vi "AutoBike FPGA backup.vi"() -> ()   [LabVIEW 2016]
doc: "The roboRIO FPGA Shipping Personality. This personality supports:\n- 8 Analog Input channels with 1 sample\n- 2 Analog Output channels with 1 sample\n- 30 Digital I/O channels with 1 sample\n- 1 RSL channel\n- 4 Relay channels\n- 1 Button\n- 3 LEDs\n- 1 Accelerometer\n- 13 PWM channels\n- 6 Encoder channels\n- 2 SPI channels\n- 2 I2C channels\n- 2 UART channels\n- 1 CAN channel\n- 2 Analog Input Interrupt\n- 5 Digital Input Interrupt\n- 1 Timer Interrupt"
uses:
  Sub VIs/Utilities/Start Boolean.ctl
  <vilib>/Platform/TimedLoop/XDataNode/timing_clust.ctl
  <vilib>/Platform/TimedLoop/XDataNode/nitl_modes.ctl
  <vilib>/Platform/TimedLoop/XDataNode/wakeup.ctl
  <vilib>/rvi/Emulation/niFpgaGetClockAttributes.vi
  <vilib>/rvi/Emulation/niFpgaSctlEmulationGetInTimedLoop.vi
  <vilib>/rvi/Emulation/niFpgaEmulationReportErrorSimple.vi
  <vilib>/rvi/eio/common/nirviEmuTemplateMethod_errors.vi
  <vilib>/rvi/Emulation/niFpgaCriticalErrorInLSC.vi
  <vilib>/rvi/Emulation/niFpgaProcessEmulError.vi
  <vilib>/rvi/Emulation/niFpgaEmulationIsFPGAContextNoSignature.vi
  <vilib>/rvi/errors/niFpgaSetErrorForExecOnDevCompSimple.vi
  <vilib>/rvi/eio/common/nirviEmuReportErrorAndStop.vi
  <vilib>/rvi/DataTransferAndStorage/Container/Common/niFpgaContainerGetUniqueNameForEmu.vi
  <vilib>/rvi/FIFO/Fifo_Resource/nirvififoEmulationSetSize.vi
  <vilib>/rvi/FIFO/Fifo_Resource/nirviFifoEmulationQueueMgr.vi
  <instcachedir>/0/nirviFifoEmulationQueueMgr_E5CAEC123FF24DC58D834DCA3CDAA9B5.lvgen/nirviFifoEmulationQueueMgr_E5CAEC123FF24DC58D834DCA3CDAA9B5_002.vi
  <vilib>/Utility/error.llb/Clear Errors.vi
  <vilib>/rvi/FIFO/Fifo_Resource/nirvififoEmulationCreateLock.vi
  <vilib>/rvi/FIFO/Fifo_Resource/nirvififoEmulationObtainLock.vi
  <vilib>/rvi/FIFO/Fifo_Resource/nirvififoEmulationReleaseLock.vi
  <vilib>/rvi/occurrence/nirviWaitOnOccurrenceBase.vi
  <vilib>/rvi/errors/nirviReportUnexpectedCaseInternalError.vi
  <vilib>/rvi/errors/nirviReportUnexpectedCaseInternalError (U32).vi
  <vilib>/rvi/FIFO/Fifo_Resource/nirvififoEmulationDetermineInputValidOut.vi
  <vilib>/rvi/DataTransferAndStorage/Container/Common/niFpgaContainerSetEmuInfo.vi
  <vilib>/eio/EIONode/EIONode.xnode
  <vilib>/rvi/DataTransferAndStorage/Container/XNode/niFpgaContainer.xnode
  <vilib>/rvi/FIFO/Fifo_Resource/nirvififoEmulationRead.vi
  <vilib>/rvi/FIFO/Fifo_Resource/nirvififoEmulationWrite.vi
  <vilib>/Platform/TimedLoop/XDataNode/XDataNode.xnode
  <vilib>/rvi/LocalResourceManager/LocalResourceManager.xnode
  <vilib>/Platform/TimedLoop/XDataNode/XDNodeRunTimeDep.lvlib
panel:
  out "Position":i64
  in  "Stop encoder":bool
  in  "Reset counter":bool
  in  "Stop direction switch":bool
  in  "Switch direction":bool
  in  "Stop the walkassist mode":bool
  in  "Initiate walkassist mode":bool
  out "HallSensorValue":u8
  in  "Stop Hallsensor":bool
  out "dt":u32
  out "dt":u32
  out "DIO.SPI_CS3:0.IN":u8 format="%08b"
  in  "DIO.SPI_CS3:0.DIR":u8 format="%08b"
  in  "DIO.SPI_CS3:0.OUT":u8 format="%08b"
  in  "IRQ.TIMER.SETTIME":T1
  in  "IRQ.TIMER.WRITE":u32
  out "IRQ.TIMER.READ":u32
  in  "IRQ.DI_BTN.NO":u8
  in  "IRQ.DI_BTN.CNT":u32
  in  "IRQ.DI_BTN.FALL":bool
  in  "IRQ.DI_BTN.RISE":bool
  in  "IRQ.DI_BTN.ENA":bool
  in  "IRQ.AI_B_0.HYSTERESIS":u16=17
  in  "IRQ.AI_B_1.HYSTERESIS":u16=17
  in  "IRQ.AI_B_1.NO":u8
  in  "IRQ.AI_B_0.NO":u8
  in  "IRQ.AI_B_1.THRESHOLD":u16
  in  "IRQ.AI_B_0.THRESHOLD":u16
  in  "IRQ.AI_B_3:0.CNFG":u8 format="%.0b"
  in  "IRQ.DIO_B_0.NO":u8
  in  "IRQ.DIO_B_1.NO":u8
  in  "IRQ.DIO_B_2.NO":u8
  in  "IRQ.DIO_B_3.NO":u8
  in  "IRQ.DIO_B_3.CNT":u32
  in  "IRQ.DIO_B_2.CNT":u32
  in  "IRQ.DIO_B_1.CNT":u32
  in  "IRQ.DIO_B_0.CNT":u32
  in  "IRQ.DIO_B_7:0.FALL":u8 format="%08b"
  in  "IRQ.DIO_B_7:0.RISE":u8 format="%08b"
  in  "IRQ.DIO_B_7:0.ENA":u8 format="%08b"
  in  "SPI.SPI.IRQ.NO":u8=15
  in  "SPI.B.IRQ.NO":u8=15
  out "DIO.DIO_9:8.IN":u8 format="%08b"
  in  "ENC.DIO_3.CNFG":u8 format="%08b"
  out "ENC.DIO_3.CNTR":u32
  out "ENC.DIO_3.STAT":u8 format="%08b"
  in  "ENC.DIO_4.CNFG":u8 format="%08b"
  out "ENC.DIO_4.CNTR":u32
  out "ENC.DIO_4.STAT":u8 format="%08b"
  in  "DIO.DIO_9:8.OUT":u8 format="%08b"
  in  "DIO.DIO_9:8.DIR":u8 format="%08b"
  in  "ENC.DIO_2.CNFG":u8 format="%08b"
  out "ENC.DIO_2.CNTR":u32
  out "ENC.DIO_2.STAT":u8 format="%08b"
  out "ENC.DIO_1.STAT":u8 format="%08b"
  out "ENC.DIO_1.CNTR":u32
  in  "ENC.DIO_1.CNFG":u8 format="%08b"
  out "DIO.DIO_7:0.IN":u8 format="%08b"
  in  "SYS.SELECTDIO":u8 format="%08b"
  in  "DIO.DIO_7:0.DIR":u8 format="%08b"
  in  "DIO.DIO_7:0.OUT":u8 format="%08b"
  out "ENC.DIO_0.STAT":u8 format="%08b"
  out "ENC.DIO_0.CNTR":u32
  in  "ENC.DIO_0.CNFG":u8 format="%08b"
  out "DI.BTN":u8 format="%08b"
  in  "DO.LED 5:0":u8 format="%06b"
  in  "DO.RSL.OUT":bool
  out "SPI.SPI.STAT":u8 format="%08b"
  in  "SPI.SPI.GO":T1
  in  "SPI.SPI.CNT":u16
  in  "SPI.SPI.CNFG":u16 format="%016b"
  out "SPI.SPI.DATI":u16
  in  "SPI.SPI.DATO":u16
  out "I2C.I2C.DATI":u8
  out "I2C.I2C.STAT":u8 format="%08b"
  in  "I2C.I2C.DATO":u8
  in  "I2C.I2CADDR":u8 format="%08b"
  in  "I2C.I2C.CNTR":u8
  in  "I2C.I2C.CNTL":u8 format="%08b"
  in  "I2C.I2C.CNFG":u8 format="%08b"
  in  "I2C.I2C.GO":T1
  out "ACC.Z.VAL":u16
  out "ACC.Y.VAL":u16
  out "ACC.X.VAL":u16
  in  "DO.RELAY.OUT":u8 format="%08b"
  out "SYS.ACC.RDY":bool
  out "SYS.RDY":bool
  in  "PWM.PWM_5.MAX":u16
  in  "PWM.PWM_5.CMP":u16
  in  "PWM.PWM_5.CNFG":u8 format="%08b"
  in  "PWM.PWM_5.CS":u8
  out "PWM.PWM_5.CNTR":u16
  in  "PWM.PWM_6.MAX":u16
  in  "PWM.PWM_6.CMP":u16
  in  "PWM.PWM_6.CNFG":u8 format="%08b"
  in  "PWM.PWM_6.CS":u8
  out "PWM.PWM_6.CNTR":u16
  in  "PWM.PWM_7.MAX":u16
  in  "PWM.PWM_7.CMP":u16
  in  "PWM.PWM_7.CNFG":u8 format="%08b"
  in  "PWM.PWM_7.CS":u8
  out "PWM.PWM_7.CNTR":u16
  in  "PWM.PWM_8.MAX":u16
  in  "PWM.PWM_8.CMP":u16
  in  "PWM.PWM_8.CNFG":u8 format="%08b"
  in  "PWM.PWM_8.CS":u8
  out "PWM.PWM_8.CNTR":u16
  in  "PWM.PWM_9.MAX":u16
  in  "PWM.PWM_9.CMP":u16
  in  "PWM.PWM_9.CNFG":u8 format="%08b"
  in  "PWM.PWM_9.CS":u8
  out "PWM.PWM_9.CNTR":u16
  in  "PWM.PWM_4.MAX":u16
  in  "PWM.PWM_4.CMP":u16
  in  "PWM.PWM_4.CNFG":u8 format="%08b"
  in  "PWM.PWM_4.CS":u8
  out "PWM.PWM_4.CNTR":u16
  in  "PWM.PWM_3.MAX":u16
  in  "PWM.PWM_3.CMP":u16
  in  "PWM.PWM_3.CNFG":u8 format="%08b"
  in  "PWM.PWM_3.CS":u8
  out "PWM.PWM_3.CNTR":u16
  in  "PWM.PWM_2.MAX":u16
  in  "PWM.PWM_2.CMP":u16
  in  "PWM.PWM_2.CNFG":u8 format="%08b"
  in  "PWM.PWM_2.CS":u8
  out "PWM.PWM_2.CNTR":u16
  in  "PWM.PWM_1.MAX":u16
  in  "PWM.PWM_1.CMP":u16
  in  "PWM.PWM_1.CNFG":u8 format="%08b"
  in  "PWM.PWM_1.CS":u8
  out "PWM.PWM_1.CNTR":u16
  out "PWM.PWM_0.CNTR":u16
  in  "PWM.PWM_0.CS":u8
  in  "PWM.PWM_0.CNFG":u8 format="%08b"
  in  "PWM.PWM_0.CMP":u16
  in  "PWM.PWM_0.MAX":u16
  in  "AO.B_0.VAL":u16
  in  "AO.B_1.VAL":u16
  in  "AO.SYS.GO":T1
  out "AO.SYS.STAT":bool
  out "AI.B_0.VAL":u16
  out "AI.B_1.VAL":u16
  out "AI.B_2.VAL":u16
  out "AI.B_3.VAL":u16
  out "AI.AI_0.VAL":u16
  out "AI.AI_1.VAL":u16
  out "AI.AI_2.VAL":u16
  out "AI.AI_3.VAL":u16
  out "SYS.AI.RDY":bool
  in  "SYS.SELECTB":u8 format="%08b"
  in  "DIO.B_7:0.OUT":u8 format="%08b"
  in  "DIO.B_7:0.DIR":u8 format="%08b"
  out "DIO.B_7:0.IN":u8 format="%08b"
  in  "DIO.B_15:8.OUT":u8 format="%08b"
  in  "DIO.B_15:8.DIR":u8 format="%08b"
  out "DIO.B_15:8.IN":u8 format="%08b"
  in  "SPI.B.DATO":u16
  out "SPI.B.DATI":u16
  in  "SPI.B.CNFG":u16 format="%016b"
  in  "SPI.B.CNT":u16
  in  "SPI.B.GO":T1
  out "SPI.B.STAT":u8 format="%08b"
  in  "PWM.B_0.MAX":u16
  in  "PWM.B_0.CMP":u16
  in  "PWM.B_0.CNFG":u8 format="%08b"
  in  "PWM.B_0.CS":u8
  out "PWM.B_0.CNTR":u16
  in  "PWM.B_1.CMP":u16
  in  "PWM.B_1.MAX":u16
  out "PWM.B_1.CNTR":u16
  in  "PWM.B_1.CNFG":u8 format="%08b"
  in  "PWM.B_1.CS":u8
  in  "PWM.B_2.CMP":u16
  in  "PWM.B_2.MAX":u16
  out "PWM.B_2.CNTR":u16
  in  "PWM.B_2.CNFG":u8 format="%08b"
  in  "PWM.B_2.CS":u8
  in  "I2C.B.DATO":u8
  out "I2C.B.DATI":u8
  in  "I2C.B.ADDR":u8 format="%08b"
  in  "I2C.B.CNTR":u8
  in  "I2C.B.CNTL":u8 format="%08b"
  out "I2C.B.STAT":u8 format="%08b"
  in  "I2C.B.CNFG":u8 format="%08b"
  in  "I2C.B.GO":T1
  in  "ENC.B.CNFG":u8 format="%08b"
  out "ENC.B.CNTR":u32
  out "ENC.B.STAT":u8 format="%08b"
  # "System"
  # "Onboard Devices"
  # "Connector B"
  # "DIO"
  # "SPI"
  # "PWM"
  # "I2C"
  # "AI"
  # "RELAY"
  # "RSL"
  # "Accelerometer"
  # "SPI Master"
  # "Analog Input"
  # "Analog Output"
  # "Digital I/O"
  # "Counters / PWM"
  # "Digital I/O"
  # "Encoders"
  # "IO Configuration"
  # "Buttons & LEDs"
  # "SPI CS DIO"
  # "Analog Interrupt"
  # "Digital Interrupt"
  # "Encoders"
  # "IO Configuration"
  # "Button Interrupt"
  # "I2C Master"
  # "FPGA Timer"
  # "This VI contains the default FPGA personality in addition to code that generates a sine waveform and filtered sine waveform based on parameters set by RT Main.vi. Keeping the default personality allows you to continue using the roboRIO APIs even after adding custom FPGA code."
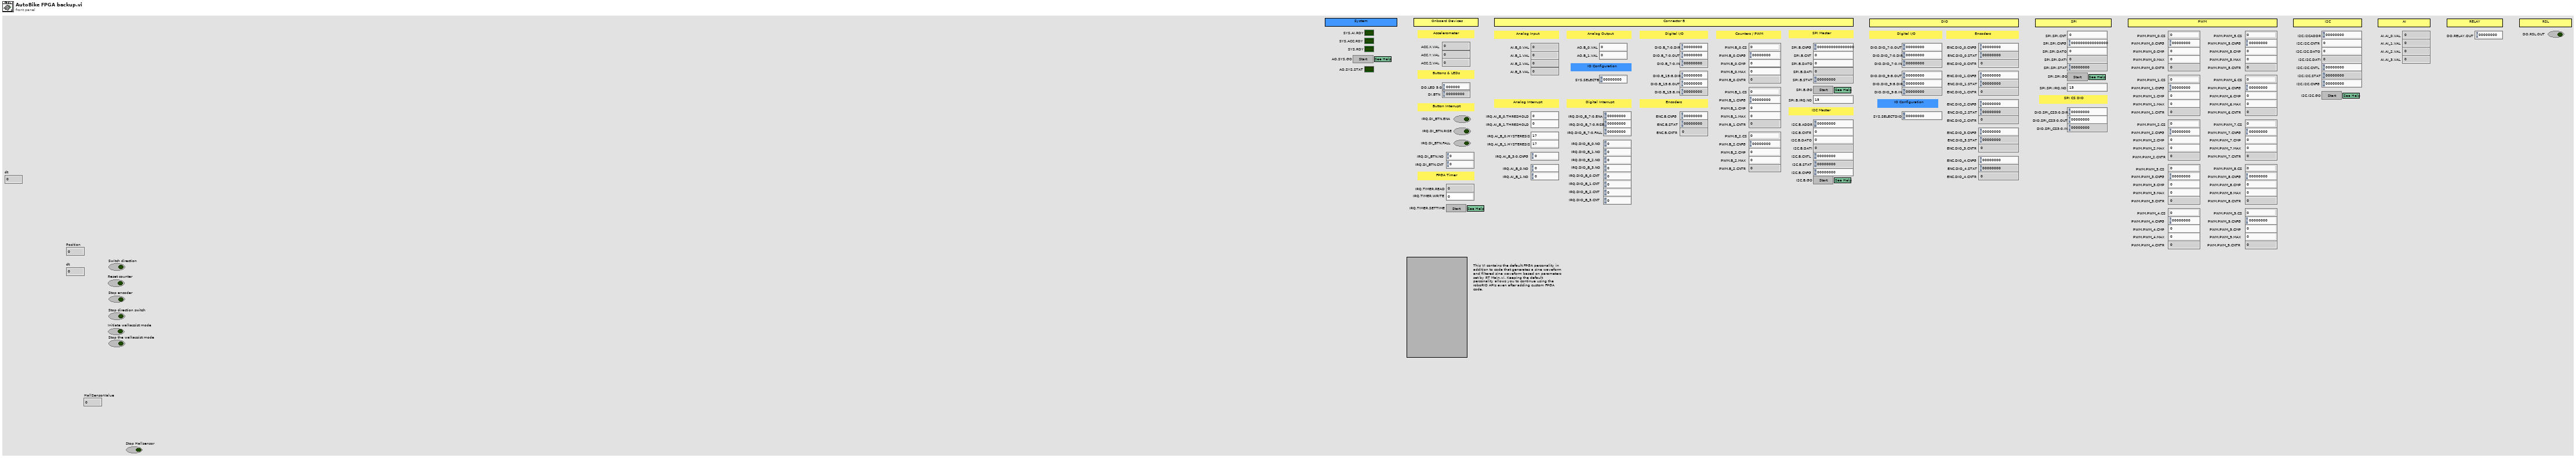
[diagram p1: front panel]
types:
  T1 = typedef "Start Boolean.ctl" = bool
  T2 = typedef "XDNodeRunTimeDep.lvlib/timing_clust.ctl" = cluster{"Expected End [f-1]":u64, "Actual End [f-1]":u64, "Finished Late? [f-1]":bool, "Expected End [i-1]":u64, "Actual End [i-1]":u64, "Finished Late? [i-1]":bool, "Expected Start [i]":u64, "Actual Start [i]":u64, "Expected Start [f]":u64, "Actual Start [f]":u64, "Source Name":string, "Structure Name":string, "Period":i64, "Deadline":i64, "Offset":i64, "Start":i64, "Priority":i32, "Timeout":i32, "Mode":T3, "Wakeup Reason":T4, "Error":errorcluster, "Source Type":string, "Secondary Source Type":string, "Global End Time":u64, "Global Start Time":u64, "Frame Duration":u64, "Iteration Duration":u64, "Assigned CPU":i32, "I/O Scan Engine Mode":u32}
  T3 = typedef "XDNodeRunTimeDep.lvlib/nitl_modes.ctl" = enum32{"No Change", "Process missed periods, maintain original phase", "Discard missed periods, maintain original phase", "Process missed periods, ignore original phase", "Discard missed periods, ignore original phase"}
  T4 = typedef "XDNodeRunTimeDep.lvlib/wakeup.ctl" = enum32{"Normal", "Aborted", "Asynchronous wakeup", "Timing source error", "Timed loop error", "Timeout"}
diagram:
  # "The accelerometer nodes take some time before the FPGA can first read the values. This is because it takes time to read from the accelerometer. An iteration of the While Loop will not complete until the accelerometer values have been read.\n\nAfter the completion of the first iteration of the While Loop, all indicators have valid values."
  # "The analog output nodes take some time before the FPGA write the values to the pins. The GO and STAT registers are used to handshake between the FPGA and host. When the host wants the values to be written, the host sets the GO register to TRUE. If the host reads the STAT register before setting the value of the GO register, it can wait for the value of the STAT register to invert. The value inversion tells the host that the output values have been written."
  # "The FPGA timer fires the interrupt request (IRQ) when TIMER.Read counts down to zero. If TIMER.Read is not zero, it counts down to one per microsecond."
  # "The analog input nodes take some time before the FPGA can first read the values. This is because it takes time to set up the Analog-to-Digital converter (ADC) and convert the first reading. An iteration of the While Loop will not complete until all the analog input channels have been sampled.\n\nAfter the completion of the first iteration of the While Loop, all indicators have valid values."
  # "Note: On some hardware a \"ghosting effect\" may occur on any unconnected AI channels. For example, if channel AI0 is connected and channels AI1~AI7 are not connected the the value read at AI0 may be seen on indicators AI1~AI7. This is common for hardware that use a multiplexed (MUXed) Analog-to-Digital converter (ADC), because the input analog signal is used to charge a capacitor which does not discharge before the unconnected channel is read.\n\nYou can hide the \"ghosting effect\" by using an mask register. This register is used to decide when the indicator should be updated."
  # "The only interface that sends interrupts to the RT side. Timer interrupts, analog input interrupts, digital input interrupts, and SPI interrupt share this interface.\n\nAll interrupts work in sequence. One interrupt waits until the previous interrupt request (IRQ) gets acknowledged on the RT side."
  # "NOTE: The SYS.RDY boolean MUST exist and must become TRUE at some point otherwise the myRIO API will not function correctly."
  # "There is some delay between when the FPGA code starts and the analog inputs, accelerometer, and scaling values outputs are valid. If the host wants to ensure that there are valid values in theses registers it should wait for each subsystem to finish its initialization process. \n\nWhen all subsystems have finished initializinig, the SYS.RDY indicator will be true, which can be polled by the host to determine the status of the FPGA. Alternatively, the host can poll the individual SYS.xx.RDY indicators to determine the status of the individual subsystems.\n\nThis loop continues indefinitely, essentially making SYS.RDY a read-only register."
  n1 = flat-sequence {
    tunnel: [i64 0] -> w3
    tunnel: [FALSE ("DIO/DIO3")] -> w2
    tunnel: [u8 0] -> w1
    tunnel: w3 -> [w34]
    tunnel: w2 -> [w33]
    tunnel: w1 -> [w28]
    frame #0 {
      # "Initialise"
    }
    frame #1 {
      n2 = while {
        shift-right: [w52] -> _
        shift-left: w33 -> [w56]
        tunnel: w28 -> [w49]
        stop <- "Stop Hallsensor" stop-if-true
        n3 = node-c288() -> (w51:T2)  [unwired: 1 in]
        n4 = call "Tick Count4"() -> ("Tick Count(uSec)"=w55:u32)
        n5 = timed-loop {
          shift-right: [w62] -> _
          shift-left: w49 -> [w73]
          tunnel: w55 -> [w71]
          shift-right: [w69] -> w52
          shift-left: w56 -> [w74]
          tunnel: [w72] -> w58
          tunnel: [w71] -> w57
          timing: w51 -> [_]
          timing-out: [_] -> w50
          i -> [w60]
          stop <- w61 stop-if-true
          # "Calculates the time it takes to collect 4 rises, i.e one revolution of the wheel"
          # "If A is high and we have a change we \nshould increament the counter"
          # "Reads the output from the hallsensor and outputs the number of change in rises"
          # "Hallsensor counter"
          n6 = call "Tick Count3"() -> ("Tick Count(uSec)"=w72:u32)
          n7 = xnode "FPGA I/O Node"() -> ("DIO/DIO3"=w69:bool)  [unwired: 1 in, 1 out]
          n8 = Equal To 0?(x=w60) -> (x = 0?=w59:bool)
          n9 = Exclusive Or(1:w74, 2:w69) -> (0:w67:bool)
          n10 = Select(t=u8 0, s=w59, f=w73) -> (s? t:f=w64:u8)
          n11 = And(x=w69, y=TRUE) -> (x .and. y?=w68:bool)
          n12 = And(x=w68, y=w67) -> (x .and. y?=w66:bool)
          n13 = Increment(x=w64) -> (x+1=w65:u8)
          n14 = Select(t=w65, s=w66, f=w64) -> (s? t:f=w62:u8)
          "HallSensorValue" <- w62
          n15 = Equal?(x=u8 4, y=w62) -> (x = y?=w61:bool)
        }
        n16 = node-c288(w50) -> ()
        n17 = Subtract(x=w58, y=w57) -> (x-y=→"dt":u32)
      }
      n18 = node-c288() -> (w30:T2)  [unwired: 1 in]
      n19 = node-c288() -> (w36:T2)  [unwired: 1 in]
      n20 = timed-loop {
        timing: w30 -> [_]
        timing-out: [_] -> w29
        stop <- "Stop the walkassist mode" stop-if-true
        # "Put the bike in walk assist."
        # "Walkassist"
        n21 = xnode "FPGA I/O Node"("DIO/DIO2"="Initiate walkassist mode") -> ()  [unwired: 1 in, 1 out]
      }
      n22 = timed-loop {
        shift-right: [w90] -> _
        shift-left: w34 -> [w81]
        shift-right: [w87] -> _
        shift-left: _ -> [w85]
        shift-right: [w86] -> _
        shift-left: _ -> [w84]
        timing: w36 -> [_]
        timing-out: [_] -> w35
        stop <- "Stop encoder" stop-if-true
        # "Decoder, reads both signals and check if there is any change to any of the channels, if there is a change current A channel\nis compared to previous B channel to determine which direction the motor is going and updates the position counter\naccordingly. The counter is resetted each time the Main VI is deployed."
        # "Motor Decoder"
        n23 = xnode "FPGA I/O Node"() -> ("DIO/DIO7"=w87:bool, "DIO/DIO8"=w86:bool)  [unwired: 2 in, 2 out]
        n24 = Exclusive Or(1:w84, 2:w87) -> (0:w83:bool)
        n25 = Select(t=i64 0, s="Reset counter", f=w81) -> (s? t:f=w89:i64)
        n26 = Exclusive Or(1:w85, 2:w87) -> (0:w97:bool)
        n27 = Exclusive Or(1:w84, 2:w86) -> (0:w96:bool)
        n28 = Or(x=w97, y=w96) -> (x .or. y?=w82:bool)
        n29 = Select(t=i64 1, s=w83, f=i64 -1) -> (s? t:f=w92:i64)
        n30 = Add(x=w92, y=w89) -> (x+y=w91:i64)
        n31 = Select(t=w91, s=w82, f=w89) -> (s? t:f=w90:i64)
        "Position" <- w90
      }
      n32 = node-c288(w29) -> ()
      n33 = node-c288() -> (w32:T2)  [unwired: 1 in]
      n34 = timed-loop {
        timing: w32 -> [_]
        timing-out: [_] -> w31
        stop <- "Stop direction switch" stop-if-true
        # "Switch the direction of the steering\nmotor."
        # "Switch direction"
        n35 = xnode "FPGA I/O Node"("DIO/DIO9"="Switch direction") -> ()  [unwired: 1 in, 1 out]
      }
      n36 = node-c288(w31) -> ()
      n37 = node-c288(w35) -> ()
    }
  }
  n38 = while {
    stop <- FALSE stop-if-true
    # "Host Synchronization"
    n39 = local read "SYS.ACC.RDY"() -> (w103:bool)
    n40 = local read "SYS.AI.RDY"() -> (w105:bool)
    n41 = Compound Arithmetic op=AND(w105, w103) -> (→"SYS.RDY":bool)
  }
  n42 = while {
    stop <- FALSE stop-if-true
    # "Interrupt to RT"
    n43 = xnode ("FIFO Method Node")("Timeout"=-1) -> ("Element"=w108:u8)  [unwired: 1 in, 2 out]
    n44 = call <vilib>:"niFPGA Interrupt.vi"("Wait Until Cleared (F)"=TRUE, "IRQ Number (0)"=w108) -> ()  [unwired: 1 in]
  }
  n45 = while {
    stop <- FALSE stop-if-true
    # "Timer"
    n46 = local read "IRQ.TIMER.READ"() -> (w113:u32)
    n47 = Select(t="IRQ.TIMER.WRITE", s="IRQ.TIMER.SETTIME", f=w113) -> (s? t:f=w111:u32)
    n48 = case shown="Default" w111 {
      selector: w111 -> [w117 w120]
      tunnel: [w117 w118] -> w110
      frame 0 {
      }
      frame Default {
        n49 = Decrement(x=w120) -> (x-1=w119:u32)
        n50 = case shown="0" w119 {
          selector: w119 -> [w121 w124]
          tunnel: [w121 w124] -> w118
          frame Default {
          }
          frame 0 {
            w123 = u8 0  # Reserved for Timer IRQ
            n51 = xnode ("FIFO Method Node")("Element"=w123, "Timeout"=-1) -> ()  [unwired: 1 in, 2 out]
          }
        }
      }
    }
    "IRQ.TIMER.READ" <- w110
    n52 = call "Loop Timer"("Count(uSec)"=u8 1 ("Count(mSec)")) -> ()  [unwired: 1 out]
  }
  n53 = xnode "VI-Defined FIFO Configuration"() -> ("FIFO Out"=w5:refnum<k21>)
  n54 = while {
    tunnel: w5 -> [w133]
    i -> [w147]
    stop <- FALSE stop-if-true
    # "Analog Input"
    n55 = Greater Than 0?(x=w147) -> (x > 0?=→"SYS.AI.RDY":bool)
    n56 = xnode "FPGA I/O Node"() -> ("MXP/AI0"=w126:u16, "MXP/AI1"=w125:u16, "MXP/AI2"=→"AI.B_2.VAL":u16, "MXP/AI3"=→"AI.B_3.VAL":u16, "AnalogIn0"=→"AI.AI_0.VAL":u16, "AnalogIn1"=→"AI.AI_1.VAL":u16, "AnalogIn2"=→"AI.AI_2.VAL":u16, "AnalogIn3"=→"AI.AI_3.VAL":u16)  [unwired: 8 in, 8 out]
    "AI.B_0.VAL" <- w126
    "AI.B_1.VAL" <- w125
    n57 = Number To Boolean Array(number="IRQ.AI_B_3:0.CNFG") -> (Boolean array=w134:bool[])
    n58 = Index Array(array=w134) -> (element #1=w136:bool, element #2=w137:bool, element #3=w139:bool, element #4=w140:bool)  [unwired: 4 in]
    n59 = call "Check AI IRQ.vi"("Hysteresis"="IRQ.AI_B_1.HYSTERESIS", "FIFO In"=w133, "IRQ Number"="IRQ.AI_B_1.NO", "Threshold"="IRQ.AI_B_1.THRESHOLD", "Analog Value"=w125, "Rising Edge?"=w140, "Enable Interrupt?"=w139) -> ()  [unwired: 5 in]
    n60 = call "Check AI IRQ.vi"("Hysteresis"="IRQ.AI_B_0.HYSTERESIS", "FIFO In"=w133, "IRQ Number"="IRQ.AI_B_0.NO", "Threshold"="IRQ.AI_B_0.THRESHOLD", "Analog Value"=w126, "Rising Edge?"=w137, "Enable Interrupt?"=w136) -> ()  [unwired: 5 in]
  }
  n61 = while {
    stop <- FALSE stop-if-true
    # "Analog Output"
    n62 = feedback #1(FALSE) -> (w151:bool)
    n63 = case shown="True" "AO.SYS.GO" {
      tunnel: "AO.B_0.VAL" -> [_ w161]
      tunnel: "AO.B_1.VAL" -> [_ w160]
      tunnel: w151 -> [w156 w159]
      tunnel: [w156 w157] -> w149
      frame False {
      }
      frame True {
        n64 = flat-sequence {
          tunnel: w161 -> [w164]
          tunnel: w160 -> [w163]
          tunnel: w159 -> [w162]
          tunnel: [w162] -> w158
          tunnel: w158 -> [w166]
          tunnel: [w165] -> w157
          frame #0 {
            n65 = xnode "FPGA I/O Node"("MXP/AO0"=w164, "MXP/AO1"=w163) -> ()  [unwired: 2 in, 2 out]
          }
          frame #1 {
            n66 = Not(x=w166) -> (.not. x?=w165:bool)
          }
        }
      }
    }
    "AO.SYS.STAT" <- w149
    n67 = feedback-in #1(w149) -> ()
  }
  n68 = while {
    i -> [w174]
    stop <- FALSE stop-if-true
    # "Onboard Accelerometer"
    n69 = xnode "FPGA I/O Node"() -> ("AccelerationX"=w172:i16, "AccelerationY"=w171:i16, "AccelerationZ"=w170:i16)  [unwired: 3 in, 3 out]
    n70 = Greater Than 0?(x=w174) -> (x > 0?=→"SYS.ACC.RDY":bool)
    n71 = To Unsigned Word Integer(number=w172) -> (unsigned 16bit integer=→"ACC.X.VAL":u16)
    n72 = To Unsigned Word Integer(number=w171) -> (unsigned 16bit integer=→"ACC.Y.VAL":u16)
    n73 = To Unsigned Word Integer(number=w170) -> (unsigned 16bit integer=→"ACC.Z.VAL":u16)
  }
  n74 = xnode "VI-Defined FIFO Configuration"() -> ("FIFO Out"=w4:refnum<k21>)
  n75 = node-c288() -> (w10:T2)  [unwired: 1 in]
  n76 = timed-loop {
    timing: w10 -> [_]
    timing-out: [_] -> w9
    tunnel: w4 -> [w181]
    stop <- FALSE stop-if-true
    # "Button IRQ"
    # "Onboard DIO"
    n77 = xnode "FPGA I/O Node"() -> ("User Button"=w182:bool)  [unwired: 1 in, 1 out]
    n78 = Number To Boolean Array(number="DO.LED 5:0") -> (Boolean array=w192:bool[])
    n79 = Index Array(array=w192) -> (element #1=w190:bool, element #2=w189:bool, element #3=w188:bool, element #4=w187:bool, element #5=w186:bool, element #6=w185:bool)  [unwired: 6 in]
    n80 = Build Array(w182) -> (w184:bool[])
    n81 = call "DIO IRQ 1-bit.vi"("IRQ.NO"="IRQ.DI_BTN.NO", "IRQ.CNT"="IRQ.DI_BTN.CNT", "FIFO in"=w181, "IRQ.FALL"="IRQ.DI_BTN.FALL", "IRQ.RISE"="IRQ.DI_BTN.RISE", "IRQ.ENA"="IRQ.DI_BTN.ENA", "DIO"=w182) -> ()  [unwired: 5 in]
    n82 = Boolean Array To Number(Boolean array=w184) -> (number=→"DI.BTN":u8)
    n83 = xnode "FPGA I/O Node"("Radio LED Green"=w190, "Radio LED Red"=w189, "Comm LED Green"=w188, "Comm LED Red"=w187, "Mode LED Green"=w186, "Mode LED Red"=w185) -> ()  [unwired: 6 in, 6 out]
  }
  n84 = while {
    stop <- FALSE stop-if-true
    # "Button SCTL Interrupt Buffer"
    n85 = feedback #2(u8 0 ("Element")) -> (w198:u8)
    n86 = feedback #3(FALSE ("Timed Out?")) -> (w202:bool)
    n87 = case shown="False" w202 {
      tunnel: [w204 w206] -> w199
      tunnel: w198 -> [_ w206]
      frame False {
        n88 = xnode ("FIFO Read")("Timeout"=-1) -> ("Element"=w204:u8)  [unwired: 1 in, 2 out]
      }
      frame True {
      }
    }
    n89 = feedback-in #2(w199) -> ()
    n90 = xnode ("FIFO Method Node")("Element"=w199, "Timeout"=0) -> ("Timed Out?"=w200:bool)  [unwired: 1 in, 1 out]
    n91 = feedback-in #3(w200) -> ()
  }
  n92 = node-c288(w9) -> ()
  n93 = xnode "VI-Defined FIFO Configuration"() -> ("FIFO Out"=w8:refnum<k21>)
  n94 = xnode "VI-Defined FIFO Configuration"() -> ("FIFO Out"=w6:refnum<k21>)
  n95 = node-c288() -> (w24:T2)  [unwired: 1 in]
  n96 = timed-loop {
    timing: w24 -> [_]
    timing-out: [_] -> w23
    tunnel: w8 -> [w243]
    tunnel: w6 -> [w231]
    stop <- _ stop-if-true
    # "DIO/ IRQ"
    # "DIO / Encoder"
    # "DIO / I2C Master"
    # "DIO / PWM"
    # "DIO"
    # "DIO"
    # "DIO/ SPI Master"
    # "Connector MXP DIO"
    n97 = call "Split HDC Bank1 DIO.vi"("IN 7:0"="DIO.B_7:0.OUT") -> ("OUT 3:0"=w331:fxp<+,4,4>, "OUT 4"=w246:bool, "OUT 7:5"=w328:fxp<+,3,3>)
    n98 = call "Split HDC Bank1 DIO.vi"("IN 7:0"="DIO.B_7:0.DIR") -> ("OUT 3:0"=w330:fxp<+,4,4>, "OUT 4"=w329:bool, "OUT 7:5"=w327:fxp<+,3,3>)
    n99 = call "Split HDC Function Select.vi"("IN 7:0"="SYS.SELECTB") -> ("OUT 1:0"=w267:fxp<+,2,2>, "OUT 7"=w262:bool, "OUT 2"=w266:bool, "OUT 3"=w265:bool, "OUT 4"=w264:bool, "OUT 5"=w263:bool)
    n100 = call "DIO 4-bit.vi"("DIO0 Refnum"=refnum<k21> "MXP/DIO0", "DIO1 Refnum"=refnum<k21> "MXP/DIO1", "DIO2 Refnum"=refnum<k21> "MXP/DIO2", "DIR 3:0"=w330, "OUT 3:0"=w331, "DIO3 Refnum"=refnum<k21> "MXP/DIO3") -> ("IN 3:0"=w242:fxp<+,4,4>)  [unwired: 5 in]
    n101 = call "DIO 1-bit.vi"("DIR"=w329, "OUT"=w246, "DIO Refnum"=refnum<k21> "MXP/DIO4") -> ("IN"=w303:bool)  [unwired: 8 in]
    n102 = call "DIO_SPI.vi"("DIO.2:0.OUT"=w328, "DIO.2:0.DIR"=w327, "SPI.CNT"="SPI.B.CNT", "SPI.CNFG"="SPI.B.CNFG", "SPI.DATO"="SPI.B.DATO", "SPI.GO"="SPI.B.GO", "DIO.2/SPI.MOSI Refnum"=refnum<k21> "MXP/DIO7" ("DIO.2/SPI.SCLK"), "SELECT.1:0"=w267, "DIO.1/SPI.MISO Refnum"=refnum<k21> "MXP/DIO6" ("DIO.1/SPI.MOSI"), "DIO.0/SPI.SCLK Refnum"=refnum<k21> "MXP/DIO5" ("DIO.0/SPI.MISO")) -> ("DIO.2:0.IN"=w302:fxp<+,3,3>, "SPI.DATI"=→"SPI.B.DATI":u16, "SPI.STAT"=w245:u8)  [unwired: 7 in]
    "SPI.B.STAT" <- w245
    n103 = call "SPI IRQ.vi"("SPI.A.IRQ.NO"="SPI.B.IRQ.NO", "SPI.STAT"=w245, "FIFO In"=w243) -> ()  [unwired: 9 in]
    n104 = call "Join HDC Bank1 DIO.vi"("IN 7:5"=w302, "IN 4"=w303, "IN 3:0"=w242) -> ("OUT 7:0"=→"DIO.B_7:0.IN":u8)
    n105 = Number To Boolean Array(number="IRQ.DIO_B_7:0.ENA") -> (Boolean array=w228:bool[])
    n106 = Number To Boolean Array(number="IRQ.DIO_B_7:0.RISE") -> (Boolean array=w219:bool[])
    n107 = Number To Boolean Array(number="IRQ.DIO_B_7:0.FALL") -> (Boolean array=w214:bool[])
    n108 = Index Array(array=w228) -> (element #1=w229:bool, element #2=w227:bool, element #3=w226:bool, element #4=w225:bool)  [unwired: 4 in]
    n109 = Index Array(array=w219) -> (element #1=w218:bool, element #2=w220:bool, element #3=w221:bool, element #4=w222:bool)  [unwired: 4 in]
    n110 = Index Array(array=w214) -> (element #1=w215:bool, element #2=w213:bool, element #3=w212:bool, element #4=w211:bool)  [unwired: 4 in]
    n111 = Build Array(w229, w227, w226, w225) -> (w230:bool[])
    n112 = Build Array(w218, w220, w221, w222) -> (w217:bool[])
    n113 = Build Array(w215, w213, w212, w211) -> (w216:bool[])
    n114 = Build Array("IRQ.DIO_B_0.CNT", "IRQ.DIO_B_1.CNT", "IRQ.DIO_B_2.CNT", "IRQ.DIO_B_3.CNT") -> (w237:u32[])
    n115 = Build Array("IRQ.DIO_B_0.NO", "IRQ.DIO_B_1.NO", "IRQ.DIO_B_2.NO", "IRQ.DIO_B_3.NO") -> (w232:u8[])
    n116 = Boolean Array To Number(Boolean array=w230) -> (number=w223:fxp<+,4,4>)
    n117 = Boolean Array To Number(Boolean array=w217) -> (number=w208:fxp<+,4,4>)
    n118 = Boolean Array To Number(Boolean array=w216) -> (number=w207:fxp<+,4,4>)
    n119 = call "DIO IRQ 4-bit.vi"("IRQ NO"=w232, "IRQ CNT"=w237, "FIFO In"=w231, "IRQ.FALL"=w207, "IRQ.RISE"=w208, "IRQ.ENA"=w223, "IN 3:0"=w242) -> ()  [unwired: 5 in]
    n120 = call "Split HDC Bank2 DIO.vi"("IN 7:0"="DIO.B_15:8.OUT") -> ("OUT 5"=w248:bool, "OUT 7:6"=w272:fxp<+,2,2>, "OUT 4:3"=w250:fxp<+,2,2>, "OUT 2"=w252:bool, "OUT 0"=w256:bool, "OUT 1"=w255:bool)  [unwired: 2 in]
    n121 = call "Split HDC Bank2 DIO.vi"("IN 7:0"="DIO.B_15:8.DIR") -> ("OUT 5"=w247:bool, "OUT 7:6"=w271:fxp<+,2,2>, "OUT 4:3"=w249:fxp<+,2,2>, "OUT 2"=w251:bool, "OUT 0"=w254:bool, "OUT 1"=w253:bool)  [unwired: 2 in]
    n122 = call "DIO_PWM.vi"("DIO.OUT"=w256, "DIO.DIR"=w254, "PWM.CS"="PWM.B_0.CS", "PWM.CNFG"="PWM.B_0.CNFG", "PWM.CMP"="PWM.B_0.CMP", "PWM.MAX"="PWM.B_0.MAX", "DIO/PWM"=refnum<k21> "MXP/DIO8", "SELECT"=w266) -> ("DIO.IN"=w261:bool, "PWM.CNTR"=→"PWM.B_0.CNTR":u16)  [unwired: 10 in]
    n123 = call "DIO_PWM.vi"("DIO.OUT"=w255, "DIO.DIR"=w253, "PWM.CS"="PWM.B_1.CS", "PWM.CNFG"="PWM.B_1.CNFG", "PWM.CMP"="PWM.B_1.CMP", "PWM.MAX"="PWM.B_1.MAX", "DIO/PWM"=refnum<k21> "MXP/DIO9", "SELECT"=w265) -> ("DIO.IN"=w260:bool, "PWM.CNTR"=→"PWM.B_1.CNTR":u16)  [unwired: 10 in]
    n124 = call "DIO_PWM.vi"("DIO.OUT"=w252, "DIO.DIR"=w251, "PWM.CS"="PWM.B_2.CS", "PWM.CNFG"="PWM.B_2.CNFG", "PWM.CMP"="PWM.B_2.CMP", "PWM.MAX"="PWM.B_2.MAX", "DIO/PWM"=refnum<k21> "MXP/DIO10", "SELECT"=w264) -> ("DIO.IN"=w259:bool, "PWM.CNTR"=→"PWM.B_2.CNTR":u16)  [unwired: 10 in]
    n125 = call "DIO_Encoder.vi"("DIO.1:0.OUT"=w250, "DIO.1:0.DIR"=w249, "QE.CNFG"="ENC.B.CNFG", "DIO.1/QE.B"=refnum<k21> "MXP/DIO12", "SELECT"=w263, "DIO.0/QE.A"=refnum<k21> "MXP/DIO11") -> ("DIO.1:0.IN"=w258:fxp<+,2,2>, "QE.CNTR"=→"ENC.B.CNTR":u32, "QE.STAT"=→"ENC.B.STAT":u8)  [unwired: 11 in]
    n126 = call "DIO 1-bit.vi"("DIR"=w247, "OUT"=w248, "DIO Refnum"=refnum<k21> "MXP/DIO13") -> ("IN"=w257:bool)  [unwired: 8 in]
    n127 = call "DIO_I2C.vi"("DIO.1:0.OUT"=w272, "DIO.1:0.DIR"=w271, "I2C.CNFG"="I2C.B.CNFG", "I2C.CNTL"="I2C.B.CNTL", "I2C.ADDR"="I2C.B.ADDR", "I2C.DATO"="I2C.B.DATO", "DIO.1/I2C.SDA"=refnum<k21> "MXP/DIO15" ("DIO.1/I2C.SCL"), "I2C.CNTR"="I2C.B.CNTR", "DIO.0/I2C.SCL"=refnum<k21> "MXP/DIO14" ("DIO.0/I2C.SDA"), "Execute?"="I2C.B.GO", "SELECT"=w262) -> ("DIO.1:0.IN"=w269:fxp<+,2,2>, "I2C.DATI"=→"I2C.B.DATI":u8, "I2C.STAT"=→"I2C.B.STAT":u8)  [unwired: 6 in]
    n128 = call "Join HDC Bank2 DIO.vi"("IN 7:6"=w269, "IN 5"=w257, "IN 4:3"=w258, "IN 0"=w261, "IN 2"=w259, "IN 1"=w260) -> ("OUT 7:0"=→"DIO.B_15:8.IN":u8)  [unwired: 4 in]
  }
  n129 = while {
    stop <- FALSE stop-if-true
    # "Connector A SPI SCTL Interrupt Buffer"
    n130 = feedback #4(u8 0 ("Element")) -> (w336:u8)
    n131 = feedback #5(FALSE ("Timed Out?")) -> (w340:bool)
    n132 = case shown="False" w340 {
      tunnel: [w342 w344] -> w337
      tunnel: w336 -> [_ w344]
      frame False {
        n133 = xnode ("FIFO Method Node")("Timeout"=-1) -> ("Element"=w342:u8)  [unwired: 1 in, 2 out]
      }
      frame True {
      }
    }
    n134 = feedback-in #4(w337) -> ()
    n135 = xnode ("FIFO Method Node")("Element"=w337, "Timeout"=0) -> ("Timed Out?"=w338:bool)  [unwired: 1 in, 1 out]
    n136 = feedback-in #5(w338) -> ()
  }
  n137 = while {
    stop <- FALSE stop-if-true
    # "Connector A DIO SCTL Interrupt Buffer"
    n138 = feedback #6(u8 0 ("Element")) -> (w347:u8)
    n139 = feedback #7(FALSE ("Timed Out?")) -> (w351:bool)
    n140 = case shown="False" w351 {
      tunnel: [w353 w355] -> w348
      tunnel: w347 -> [_ w355]
      frame False {
        n141 = xnode ("FIFO Method Node")("Timeout"=-1) -> ("Element"=w353:u8)  [unwired: 1 in, 2 out]
      }
      frame True {
      }
    }
    n142 = feedback-in #6(w348) -> ()
    n143 = xnode ("FIFO Method Node")("Element"=w348, "Timeout"=0) -> ("Timed Out?"=w349:bool)  [unwired: 1 in, 1 out]
    n144 = feedback-in #7(w349) -> ()
  }
  n145 = node-c288(w23) -> ()
  n146 = node-c288() -> (w18:T2)  [unwired: 1 in]
  n147 = timed-loop {
    timing: w18 -> [_]
    timing-out: [_] -> w17
    stop <- FALSE stop-if-true
    # "DIO"
    n148 = call "Split HDC Bank3 DIO.vi"("IN 7:0"="DIO.DIO_7:0.OUT") -> ("OUT 1:0"=w371:fxp<+,2,2>, "OUT 3:2"=w370:fxp<+,2,2>, "OUT 5:4"=w369:fxp<+,2,2>, "OUT 7:6"=w361:fxp<+,2,2>)
    n149 = call "Split HDC Bank3 DIO.vi"("IN 7:0"="DIO.DIO_7:0.DIR") -> ("OUT 1:0"=w367:fxp<+,2,2>, "OUT 3:2"=w366:fxp<+,2,2>, "OUT 5:4"=w365:fxp<+,2,2>, "OUT 7:6"=w360:fxp<+,2,2>)
    n150 = Number To Boolean Array(number="SYS.SELECTDIO") -> (Boolean array=w402:bool[])
    n151 = Index Array(array=w402) -> (element #1=w401:bool, element #2=w398:bool, element #3=w389:bool, element #4=w378:bool, element #5=w377:bool)  [unwired: 5 in]
    n152 = call "DIO_Encoder.vi"("DIO.1:0.OUT"=w361, "DIO.1:0.DIR"=w360, "QE.CNFG"="ENC.DIO_3.CNFG", "DIO.1/QE.B"=refnum<k21> "DIO/DIO7" ("DIO Refnum"), "SELECT"=w378, "DIO.0/QE.A"=refnum<k21> "DIO/DIO6" ("DIO Refnum")) -> ("DIO.1:0.IN"=w359:fxp<+,2,2>, "QE.CNTR"=→"ENC.DIO_3.CNTR":u32, "QE.STAT"=→"ENC.DIO_3.STAT":u8)  [unwired: 11 in]
    n153 = call "DIO_Encoder.vi"("DIO.1:0.OUT"=w371, "DIO.1:0.DIR"=w367, "QE.CNFG"="ENC.DIO_0.CNFG", "DIO.1/QE.B"=refnum<k21> "DIO/DIO1" ("DIO Refnum"), "SELECT"=w401, "DIO.0/QE.A"=refnum<k21> "DIO/DIO0" ("DIO Refnum")) -> ("DIO.1:0.IN"=w376:fxp<+,2,2>, "QE.CNTR"=→"ENC.DIO_0.CNTR":u32, "QE.STAT"=→"ENC.DIO_0.STAT":u8)  [unwired: 11 in]
    n154 = call "DIO_Encoder.vi"("DIO.1:0.OUT"=w370, "DIO.1:0.DIR"=w366, "QE.CNFG"="ENC.DIO_1.CNFG", "DIO.1/QE.B"=refnum<k21> "DIO/DIO3" ("DIO Refnum"), "SELECT"=w398, "DIO.0/QE.A"=refnum<k21> "DIO/DIO2" ("DIO Refnum")) -> ("DIO.1:0.IN"=w375:fxp<+,2,2>, "QE.CNTR"=→"ENC.DIO_1.CNTR":u32, "QE.STAT"=→"ENC.DIO_1.STAT":u8)  [unwired: 11 in]
    n155 = call "DIO_Encoder.vi"("DIO.1:0.OUT"=w369, "DIO.1:0.DIR"=w365, "QE.CNFG"="ENC.DIO_2.CNFG", "DIO.1/QE.B"=refnum<k21> "DIO/DIO5" ("DIO Refnum"), "SELECT"=w389, "DIO.0/QE.A"=refnum<k21> "DIO/DIO4" ("DIO Refnum")) -> ("DIO.1:0.IN"=w374:fxp<+,2,2>, "QE.CNTR"=→"ENC.DIO_2.CNTR":u32, "QE.STAT"=→"ENC.DIO_2.STAT":u8)  [unwired: 11 in]
    n156 = call "Join HDC Bank3 DIO.vi"("IN 7:6"=w359, "IN 5:4"=w374, "IN 3:2"=w375, "IN 1:0"=w376) -> ("OUT 7:0"=→"DIO.DIO_7:0.IN":u8)
    n157 = call "Split HDC Bank3 DIO.vi"("IN 7:0"="DIO.DIO_9:8.OUT") -> ("OUT 1:0"=w358:fxp<+,2,2>)  [unwired: 3 out]
    n158 = call "Split HDC Bank3 DIO.vi"("IN 7:0"="DIO.DIO_9:8.DIR") -> ("OUT 1:0"=w357:fxp<+,2,2>)  [unwired: 3 out]
    n159 = call "DIO_Encoder.vi"("DIO.1:0.OUT"=w358, "DIO.1:0.DIR"=w357, "QE.CNFG"="ENC.DIO_4.CNFG", "DIO.1/QE.B"=refnum<k21> "DIO/DIO9" ("DIO Refnum"), "SELECT"=w377, "DIO.0/QE.A"=refnum<k21> "DIO/DIO8" ("DIO Refnum")) -> ("DIO.1:0.IN"=w356:fxp<+,2,2>, "QE.CNTR"=→"ENC.DIO_4.CNTR":u32, "QE.STAT"=→"ENC.DIO_4.STAT":u8)  [unwired: 11 in]
    n160 = call "Join HDC Bank3 DIO.vi"("IN 1:0"=w356) -> ("OUT 7:0"=→"DIO.DIO_9:8.IN":u8)  [unwired: 3 in]
  }
  n161 = node-c288(w17) -> ()
  n162 = node-c288() -> (w22:T2)  [unwired: 1 in]
  n163 = timed-loop {
    timing: w22 -> [_]
    timing-out: [_] -> w21
    stop <- FALSE stop-if-true
    # "PWM"
    n164 = call "PWM (Single Output).vi"("Clock Select"="PWM.PWM_0.CS", "Counter Control"="PWM.PWM_0.CNFG", "Output Compare Value"="PWM.PWM_0.CMP", "Max Counter Value"="PWM.PWM_0.MAX") -> ("Output"=w467:bool, "Counter Value"=→"PWM.PWM_0.CNTR":u16)  [unwired: 6 in]
    n165 = call "PWM (Single Output).vi"("Clock Select"="PWM.PWM_1.CS", "Counter Control"="PWM.PWM_1.CNFG", "Output Compare Value"="PWM.PWM_1.CMP", "Max Counter Value"="PWM.PWM_1.MAX") -> ("Output"=w461:bool, "Counter Value"=→"PWM.PWM_1.CNTR":u16)  [unwired: 6 in]
    n166 = call "PWM (Single Output).vi"("Clock Select"="PWM.PWM_2.CS", "Counter Control"="PWM.PWM_2.CNFG", "Output Compare Value"="PWM.PWM_2.CMP", "Max Counter Value"="PWM.PWM_2.MAX") -> ("Output"=w445:bool, "Counter Value"=→"PWM.PWM_2.CNTR":u16)  [unwired: 6 in]
    n167 = call "PWM (Single Output).vi"("Clock Select"="PWM.PWM_3.CS", "Counter Control"="PWM.PWM_3.CNFG", "Output Compare Value"="PWM.PWM_3.CMP", "Max Counter Value"="PWM.PWM_3.MAX") -> ("Output"=w444:bool, "Counter Value"=→"PWM.PWM_3.CNTR":u16)  [unwired: 6 in]
    n168 = call "PWM (Single Output).vi"("Clock Select"="PWM.PWM_4.CS", "Counter Control"="PWM.PWM_4.CNFG", "Output Compare Value"="PWM.PWM_4.CMP", "Max Counter Value"="PWM.PWM_4.MAX") -> ("Output"=w443:bool, "Counter Value"=→"PWM.PWM_4.CNTR":u16)  [unwired: 6 in]
    n169 = xnode "FPGA I/O Node"("PWM/PWM0"=w467, "PWM/PWM1"=w461, "PWM/PWM2"=w445, "PWM/PWM3"=w444, "PWM/PWM4"=w443) -> ()  [unwired: 5 in, 5 out]
    n170 = call "PWM (Single Output).vi"("Clock Select"="PWM.PWM_5.CS", "Counter Control"="PWM.PWM_5.CNFG", "Output Compare Value"="PWM.PWM_5.CMP", "Max Counter Value"="PWM.PWM_5.MAX") -> ("Output"=w418:bool, "Counter Value"=→"PWM.PWM_5.CNTR":u16)  [unwired: 6 in]
    n171 = call "PWM (Single Output).vi"("Clock Select"="PWM.PWM_6.CS", "Counter Control"="PWM.PWM_6.CNFG", "Output Compare Value"="PWM.PWM_6.CMP", "Max Counter Value"="PWM.PWM_6.MAX") -> ("Output"=w424:bool, "Counter Value"=→"PWM.PWM_6.CNTR":u16)  [unwired: 6 in]
    n172 = call "PWM (Single Output).vi"("Clock Select"="PWM.PWM_7.CS", "Counter Control"="PWM.PWM_7.CNFG", "Output Compare Value"="PWM.PWM_7.CMP", "Max Counter Value"="PWM.PWM_7.MAX") -> ("Output"=w440:bool, "Counter Value"=→"PWM.PWM_7.CNTR":u16)  [unwired: 6 in]
    n173 = call "PWM (Single Output).vi"("Clock Select"="PWM.PWM_8.CS", "Counter Control"="PWM.PWM_8.CNFG", "Output Compare Value"="PWM.PWM_8.CMP", "Max Counter Value"="PWM.PWM_8.MAX") -> ("Output"=w441:bool, "Counter Value"=→"PWM.PWM_8.CNTR":u16)  [unwired: 6 in]
    n174 = call "PWM (Single Output).vi"("Clock Select"="PWM.PWM_9.CS", "Counter Control"="PWM.PWM_9.CNFG", "Output Compare Value"="PWM.PWM_9.CMP", "Max Counter Value"="PWM.PWM_9.MAX") -> ("Output"=w442:bool, "Counter Value"=→"PWM.PWM_9.CNTR":u16)  [unwired: 6 in]
    n175 = xnode "FPGA I/O Node"("PWM/PWM5"=w418, "PWM/PWM6"=w424, "PWM/PWM7"=w440, "PWM/PWM8"=w441, "PWM/PWM9"=w442) -> ()  [unwired: 5 in, 5 out]
  }
  n176 = node-c288(w21) -> ()
  n177 = xnode "VI-Defined FIFO Configuration"() -> ("FIFO Out"=w7:refnum<k21>)
  n178 = node-c288() -> (w14:T2)  [unwired: 1 in]
  n179 = timed-loop {
    timing: w14 -> [_]
    timing-out: [_] -> w13
    tunnel: w7 -> [w477]
    stop <- FALSE stop-if-true
    # "SPI / CS DIO"
    # "SPI / SPI"
    # "SPI"
    n180 = xnode "FPGA I/O Node"() -> ("SPI MISO"=w494:bool)  [unwired: 1 in, 1 out]
    n181 = call "SPI Master.vi"("Count"="SPI.SPI.CNT", "Configuration"="SPI.SPI.CNFG", "Start?"="SPI.SPI.GO", "MISO"=w494, "Data Out"="SPI.SPI.DATO") -> ("Status"=w475:u8, "SCLK"=w488:bool, "MOSI"=w489:bool, "Data In"=→"SPI.SPI.DATI":u16)  [unwired: 3 in]
    "SPI.SPI.STAT" <- w475
    n182 = xnode "FPGA I/O Node"("SPI MOSI"=w489, "SPI CLK"=w488) -> ()  [unwired: 2 in, 2 out]
    n183 = call "SPI IRQ.vi"("SPI.A.IRQ.NO"="SPI.SPI.IRQ.NO", "SPI.STAT"=w475, "FIFO In"=w477) -> ()  [unwired: 9 in]
    n184 = call "Split HDC Bank1 DIO.vi"("IN 7:0"="DIO.SPI_CS3:0.OUT") -> ("OUT 3:0"=w484:fxp<+,4,4>)  [unwired: 2 out]
    n185 = call "Split HDC Bank1 DIO.vi"("IN 7:0"="DIO.SPI_CS3:0.DIR") -> ("OUT 3:0"=w483:fxp<+,4,4>)  [unwired: 2 out]
    n186 = call "DIO 4-bit.vi"("DIO0 Refnum"=refnum<k21> "SPI CS0", "DIO1 Refnum"=refnum<k21> "SPI CS1" ("DIO0 Refnum"), "DIO2 Refnum"=refnum<k21> "SPI CS2" ("DIO0 Refnum"), "DIR 3:0"=w483, "OUT 3:0"=w484, "DIO3 Refnum"=refnum<k21> "SPI CS3" ("DIO0 Refnum")) -> ("IN 3:0"=w482:fxp<+,4,4>)  [unwired: 5 in]
    n187 = call "Join HDC Bank1 DIO.vi"("IN 3:0"=w482) -> ("OUT 7:0"=→"DIO.SPI_CS3:0.IN":u8)  [unwired: 2 in]
  }
  n188 = while {
    stop <- FALSE stop-if-true
    # "Connector SPI SPI SCTL Interrupt Buffer"
    n189 = feedback #8(u8 0 ("Element")) -> (w501:u8)
    n190 = feedback #9(FALSE ("Timed Out?")) -> (w505:bool)
    n191 = case shown="False" w505 {
      tunnel: [w507 w509] -> w502
      tunnel: w501 -> [_ w509]
      frame False {
        n192 = xnode ("FIFO Method Node")("Timeout"=-1) -> ("Element"=w507:u8)  [unwired: 1 in, 2 out]
      }
      frame True {
      }
    }
    n193 = feedback-in #8(w502) -> ()
    n194 = xnode ("FIFO Method Node")("Element"=w502, "Timeout"=0) -> ("Timed Out?"=w503:bool)  [unwired: 1 in, 1 out]
    n195 = feedback-in #9(w503) -> ()
  }
  n196 = node-c288(w13) -> ()
  n197 = node-c288() -> (w16:T2)  [unwired: 1 in]
  n198 = timed-loop {
    timing: w16 -> [_]
    timing-out: [_] -> w15
    stop <- FALSE stop-if-true
    # "I2C"
    n199 = call "DIO_I2C.vi"("I2C.CNFG"="I2C.I2C.CNFG", "I2C.CNTL"="I2C.I2C.CNTL", "I2C.ADDR"="I2C.I2CADDR", "I2C.DATO"="I2C.I2C.DATO", "DIO.1/I2C.SDA"=refnum<k21> "I2C SDA" ("FPGA I/O In"), "I2C.CNTR"="I2C.I2C.CNTR", "DIO.0/I2C.SCL"=refnum<k21> "I2C SCL" ("FPGA I/O In"), "Execute?"="I2C.I2C.GO", "SELECT"=TRUE) -> ("I2C.DATI"=→"I2C.I2C.DATI":u8, "I2C.STAT"=→"I2C.I2C.STAT":u8)  [unwired: 8 in, 1 out]
  }
  n200 = node-c288(w15) -> ()
  n201 = node-c288() -> (w20:T2)  [unwired: 1 in]
  n202 = timed-loop {
    timing: w20 -> [_]
    timing-out: [_] -> w19
    stop <- FALSE stop-if-true
    # "Relay"
    n203 = Number To Boolean Array(number="DO.RELAY.OUT") -> (Boolean array=w532:bool[])
    n204 = Index Array(array=w532) -> (element #1=w531:bool, element #2=w530:bool, element #3=w529:bool, element #4=w528:bool, element #5=w527:bool, element #6=w526:bool, element #7=w525:bool, element #8=w524:bool)  [unwired: 8 in]
    n205 = xnode "FPGA I/O Node"("RelayFwd0"=w531, "RelayRev0"=w530, "RelayFwd1"=w529, "RelayRev1"=w528, "RelayFwd2"=w527, "RelayRev2"=w526, "RelayFwd3"=w525, "RelayRev3"=w524) -> ()  [unwired: 8 in, 8 out]
  }
  n206 = node-c288(w19) -> ()
  n207 = node-c288() -> (w12:T2)  [unwired: 1 in]
  n208 = timed-loop {
    timing: w12 -> [_]
    timing-out: [_] -> w11
    stop <- FALSE stop-if-true
    # "RSL"
    n209 = xnode "FPGA I/O Node"("RSL"="DO.RSL.OUT") -> ()  [unwired: 1 in, 1 out]
  }
  n210 = node-c288(w11) -> ()
